vi "Initialize Motion.vi"(7 "Location":T1, 8 "error in":errorcluster, 9 "Bypass Motion Init":bool, 10 "Main Digitizer":T2=enum."NI Digitizer", 11 "Motion Settings In":T3={"No Motion?"=FALSE, "Motion System"=enum."MM3000", "Motion Bd ID"=0, "Motion Profile"="SMAC1", "# Axis"=0, "Reverse Z axis?"=FALSE, "SMAC Axis"=0, "scan pair"=enum."y-(x) scan", "RT fps"=0.0, "Steps per mm"=[], "Motor Parameters"={"velocity ct/s"=[], "accel ct/s^2"=[]}, "One Way Scan"=FALSE, "Reverse One Way Scan"=FALSE, "Global Position (mm)"=[], "Plane"=0, "Distance between\nscan lines (um)"=0.0, "Distance between\nscan planes (um)"=0.0, "number of scan planes"=0, "Total steps in line"=0, "Xtra plane\ndistance  (um)"=0, "Xtra planes "=0, "Add Axis"=FALSE, "overshoot cts"=0, "BKPT Shift"=0, "Scan Start Time (ms)"=0, "ESP VISA"="", "3rd Axis"=1, "GL Ref Out"=refnum, "Galil Address"=""} {"3rd Axis" items=["x", "y", "z", "w"]; "Xtra planes" min=1; "Xtra plane\ndistance  (um)" min=0; "Distance between\nscan planes (um)" format="%.2f"; "Distance between\nscan lines (um)" format="%.2f"; "SMAC Axis" items=["None"=0, "Axis 1"=1, "Axis 2"=2, "Axis 3"=3, "Axis 4"=4, "Axis 5"=5, "Axis 6"=6, "Axis 7"=7, "Axis 8"=8, "Vector Space 1"=17, "Vector Space 2"=18, "Vector Space 3"=19, "Vector Space 4"=20]; "Motion Bd ID" min=1 max=32 step=1}) -> (0 "error out":errorcluster, 1 "Initialization Failed!!":bool, 3 "Motion Settings":T3={"No Motion?"=FALSE, "Motion System"=enum."MM3000", "Motion Bd ID"=0, "Motion Profile"="SMAC1", "# Axis"=0, "Reverse Z axis?"=FALSE, "SMAC Axis"=0, "scan pair"=enum."y-(x) scan", "RT fps"=0.0, "Steps per mm"=[], "Motor Parameters"={"velocity ct/s"=[], "accel ct/s^2"=[]}, "One Way Scan"=FALSE, "Reverse One Way Scan"=FALSE, "Global Position (mm)"=[], "Plane"=0, "Distance between\nscan lines (um)"=0.0, "Distance between\nscan planes (um)"=0.0, "number of scan planes"=0, "Total steps in line"=0, "Xtra plane\ndistance  (um)"=0, "Xtra planes "=0, "Add Axis"=FALSE, "overshoot cts"=0, "BKPT Shift"=0, "Scan Start Time (ms)"=0, "ESP VISA"="", "3rd Axis"=1, "GL Ref Out"=refnum, "Galil Address"=""} {"3rd Axis" items=["x", "y", "z", "w"]; "Xtra planes" min=1; "Xtra plane\ndistance  (um)" min=0; "Distance between\nscan planes (um)" format="%.2f"; "Distance between\nscan lines (um)" format="%.2f"; "SMAC Axis" items=["None"=0, "Axis 1"=1, "Axis 2"=2, "Axis 3"=3, "Axis 4"=4, "Axis 5"=5, "Axis 6"=6, "Axis 7"=7, "Axis 8"=8, "Vector Space 1"=17, "Vector Space 2"=18, "Vector Space 3"=19, "Vector Space 4"=20]; "Motion Bd ID" min=1 max=32 step=1})   [LabVIEW 2022 SP3]
uses:
  NI_controller/-NI_MotionRoutines/MotionParameters.ctl
  NI_controller/-NI_MotionRoutines/MotionSys.ctl
  -MotionRoutines/ScanAxis.ctl
  -MotionRoutines/3rdAxis.ctl
  Digitizers/-DigitizerRoutines/Digitizer.ctl
  -ScanSystem/Controls/location.ctl
  Galil/Command Menu.ctl
  <vilib>/DAQmx/write.llb/DAQmx Write (Digital Bool 1Line 1Point).vi
  -MotionRoutines/MotionGlobals.vi
  <vilib>/DAQmx/miscellaneous.llb/DAQmx Fill In Error Info.vi
  <instrlib>/Newport ESP301/Newport ESP301.lvlib
panel:
  # "1-D and 2-D B scan settings"
  # "1-D and 2-D B scan settings"
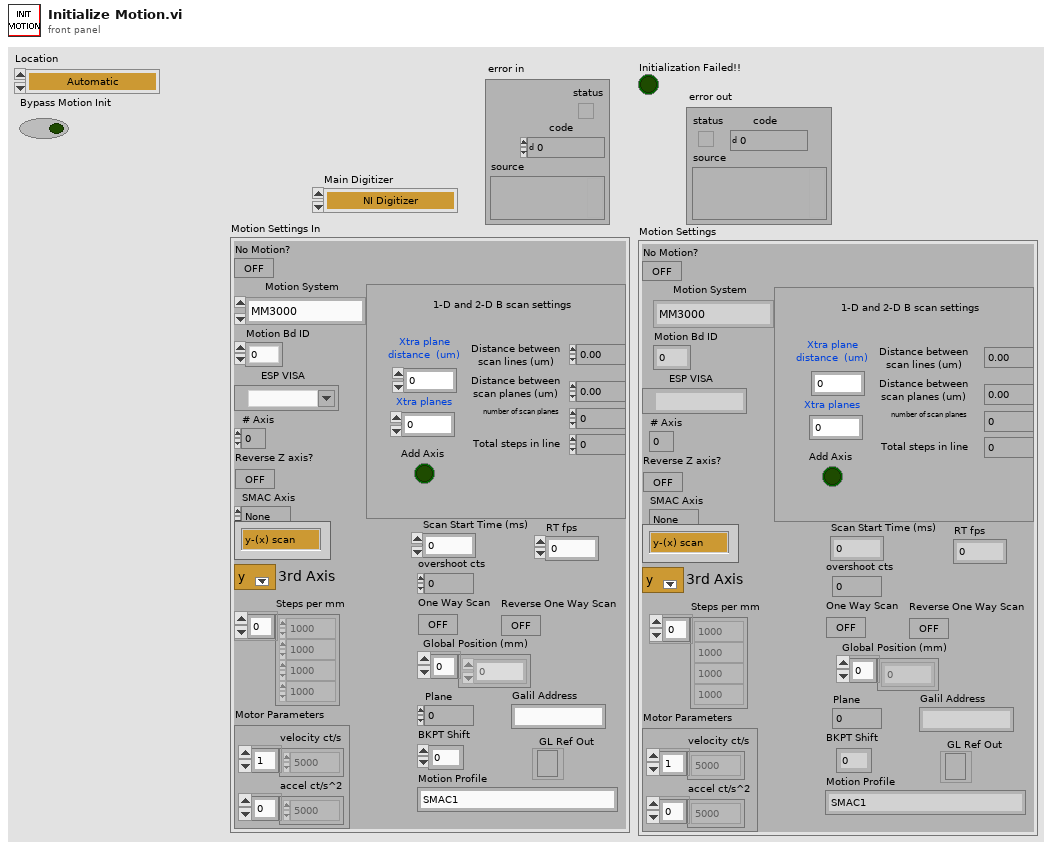
[diagram p1: front panel]
types:
  T1 = typedef "location.ctl" = enum16{"Automatic", "WCM Main", "Hawaii", "Columbia MM3000", "Columbia  NI System", "NYU", "RRI 2", "UHI Allen", "CUMC RT", "Chiba", "Stony Brook", "WCM Microscopy", "WCM Aeoretch", "WCM Optics Lab", "WCM Main 2Axis", "WCM Rotation", "WCM SAM SMAC", "SERI GP", "SERI SAM 2023"}
  T2 = typedef "Digitizer.ctl" = enum16{"Acqiris Digitizer", "NI Digitizer", "LeCroy", "GaGe", "AlazarTech", "No Digitizer", "Teledyne"}
  T3 = typedef "MotionParameters.ctl" = cluster{"No Motion?":bool, "Motion System":T4, "Motion Bd ID":u8, "Motion Profile":string, "# Axis":i8, "Reverse Z axis?":bool, "SMAC Axis":u16, "scan pair":T5, "RT fps":sgl, "Steps per mm":i32[], "Motor Parameters":cluster{"velocity ct/s":dbl[], "accel ct/s^2":dbl[]}, "One Way Scan":bool, "Reverse One Way Scan":bool, "Global Position (mm)":dbl[], "Plane":i32, "Distance between\nscan lines (um)":sgl, "Distance between\nscan planes (um)":sgl, "number of scan planes":i32, "Total steps in line":i32, "Xtra plane\ndistance  (um)":i32, "Xtra planes ":i32, "Add Axis":bool, "overshoot cts":i32, "BKPT Shift":i32, "Scan Start Time (ms)":u32, "ESP VISA":refnum<visa-resource-name>, "3rd Axis":T6, "GL Ref Out":refnum<k7>, "Galil Address":string}
  T4 = typedef "MotionSys.ctl" = enum16{"MM3000", "NI 735x", "Newport ESP", "No Motion Card", "Galil"}
  T5 = typedef "ScanAxis.ctl" = enum16{"y-(x) scan", "x-(y) scan", "z-(x) scan", "z-(y) scan", "y-(z) scan", "x-(z) scan", "w-(x) scan", "w-(y) scan", "w-(z) scan", "x-(w) scan", "y-(w) scan", "z-(w) scan"}
  T6 = typedef "3rdAxis.ctl" = u16
  T7 = cluster{"Port A (T:output, F:input)":bool, "Port B (T:output, F:input)":bool}
  T8 = typedef "Command Menu.ctl" = enum16{"CommandPassThrough", "Abort Motion", "Define Pos", "Velocity", "Acceleration", "Deceleration", "Position Rel", "Postion Abs", "Begin Move", "After Move", "Home", "KI", "KD", "KP", "IL", "Config I/O", "Set Bit", "Clear Bit", "Motor Off", "Moto On", "Status", "Execute", "Halt Execute", "HX Status", "Tell Velocity", "Check Motion", "BreakPoint", "Tell Position", "Current Code Line", "Tell Switches", "OC Force On", "OC Off", "Pos Soft Limit", "Rev Soft Limit"}
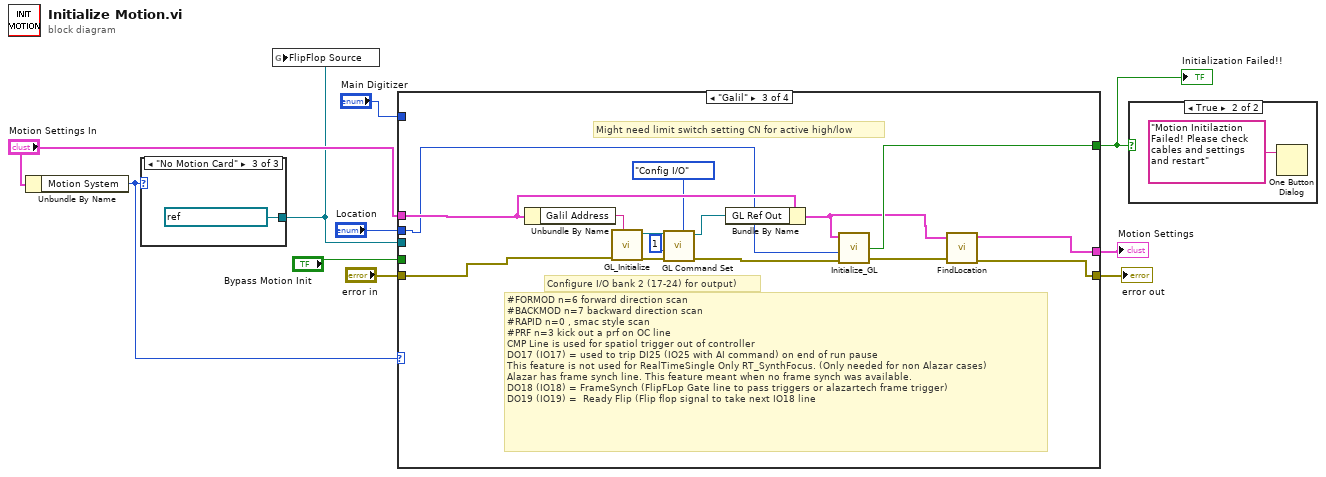
[diagram p0: block diagram]
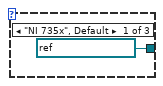
[diagram p3: hidden frame]
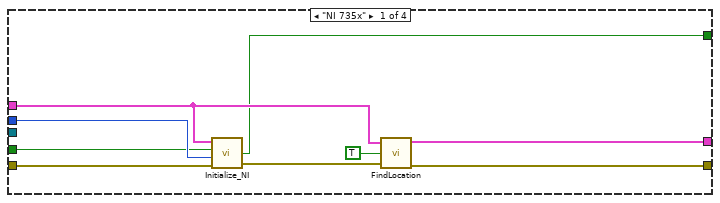
[diagram p5: hidden frame]
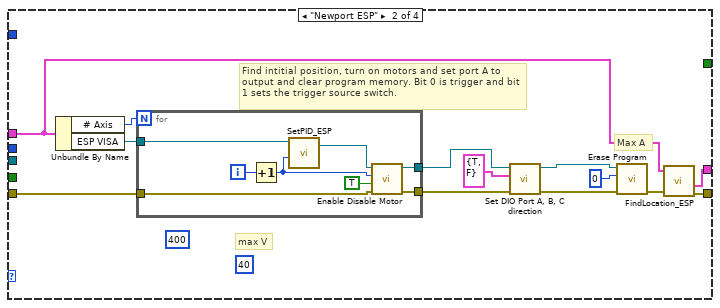
[diagram p6: hidden frame]
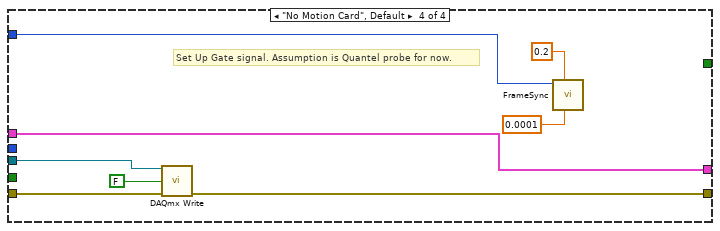
[diagram p7: hidden frame]
diagram:
  n1 = Unbundle By Name("Motion Settings In") -> ("Motion System"=w8:T4)
  n2 = case shown="\"No Motion Card\"" w8 {
    tunnel: [refnum<k21> "Dev1 FlipFlop" ("FlipFlop Source") _ refnum<k21> "QuantFlipFlop" ("FlipFlop Source")] -> w7
    frame "NI 735x", Default {
    }
    frame "Galil" {
    }
    frame "No Motion Card" {
    }
  }
  n3 = global write "MotionGlobals.vi" "FlipFlop Source"(w7) -> ()
  n4 = case shown="\"Galil\"" w8 {
    tunnel: w7 -> [_ _ _ w63]
    tunnel: "Motion Settings In" -> [w19 w26 w56 w61]
    tunnel: [w20 w28 w57 w61] -> w9
    tunnel: [w18 _ w46 _] -> w4
    tunnel: "error in" -> [w17 w22 w55 w59]
    tunnel: [w16 w24 w47 w60] -> w5
    tunnel: "Main Digitizer" -> [_ _ _ w58]
    tunnel: "Location" -> [w14 _ w54 _]
    tunnel: "Bypass Motion Init" -> [w13 _ _ _]
    frame "NI 735x" {
      n5 = call "Initialize_NI.vi"("Motion Settings"=w19, "Bypass Motion Init"=w13, "Location"=w14, "error in"=w17) -> ("Initialization Failed!!"=w18:bool, "error out"=w21:errorcluster)  [unwired: 1 in, 1 out]
      n6 = call "FindLocation.vi"("Motion Settings"=w19, "Wait for Motion Complete"=TRUE, "error in (no error)"=w21) -> ("Motion Settings Out"=w20:T3, "error out"=w16:errorcluster)  [unwired: 2 out]
    }
    frame "Newport ESP" {
      (unwired) 400
      (unwired) 40
      # "Max A"
      # "max V"
      # "Find intitial position, turn on motors and set port A to output and clear program memory. Bit 0 is trigger and bit 1 sets the trigger source switch."
      n7 = Unbundle By Name(w26) -> ("# Axis"=w25:i8, "ESP VISA"=w30:refnum<visa-resource-name>)
      n8 = for {
        N: w25 -> [_]
        tunnel: [w40] -> w29
        tunnel: w30 -> [w39]
        tunnel: [w36] -> w23
        tunnel: w22 -> [w35]
        i -> [w42]
        n9 = Increment(x=w42) -> (x+1=w37:i32)
        n10 = call "SetPID_ESP.vi"("VISA resource name"=w39, "Axis"=w37) -> ("VISA resource name out"=w38:refnum<visa-resource-name>)  [unwired: 4 in]
        n11 = call <instrlib>:"Enable Disable Motor.vi"("error in (no error)"=w35, "Action (OFF)"=TRUE, "Axis (1)"=w37, "VISA resource name"=w38) -> ("error out"=w36:errorcluster, "VISA resource name out"=w40:refnum<visa-resource-name>)  [unwired: 2 in]
      }
      n12 = call <instrlib>:"Set DIO Port A, B, C direction.vi"("error in (no error)"=w23, "Port A, B direction"=T7 {"Port A (T:output, F:input)"=TRUE, "Port B (T:output, F:input)"=FALSE}, "VISA resource name"=w29) -> ("error out"=w31:errorcluster, "VISA resource name out"=w32:refnum<visa-resource-name>)  [unwired: 7 in]
      n13 = call <instrlib>:"Erase Program.vi"("error in (no error)"=w31, "Program # (1)"=0, "VISA resource name"=w32) -> ("error out"=w27:errorcluster)  [unwired: 3 in, 1 out]
      n14 = call "FindLocation_ESP.vi"("Motion Settings"=w26, "error in (no error)"=w27) -> ("Motion Settings Out"=w28:T3, "error out"=w24:errorcluster)  [unwired: 1 in, 2 out]
    }
    frame "Galil" {
      # "Configure I/O bank 2 (17-24) for output)"
      # "#FORMOD n=6 forward direction scan\n#BACKMOD n=7 backward direction scan\n#RAPID n=0 , smac style scan\n#PRF n=3 kick out a prf on OC line\nCMP Line is used for spatiol trigger out of controller\nDO17 (IO17) = used to trip DI25 (IO25 with AI command) on end of run pause \nThis feature is not used for RealTimeSingle Only RT_SynthFocus. (Only needed for non Alazar cases)\nAlazar has frame synch line. This feature meant when no frame synch was available.\nDO18 (IO18) = FrameSynch (FlipFLop Gate line to pass triggers or alazartech frame trigger)\nDO19 (IO19) =  Ready Flip (Flip flop signal to take next IO18 line"
      # "Might need limit switch setting CN for active high/low"
      n15 = Unbundle By Name(w56) -> ("Galil Address"=w51:string)
      n16 = call "GL_Initialize.vi"("IP Address/COM"=w51, "error in (no error)"=w55) -> ("error out"=w49:errorcluster, "GL Ref Out"=w50:refnum<k7>)  [unwired: 4 in, 2 out]
      n17 = call "GL Command Set.vi"("Command"=Command_Menu."Config I/O", "error in (no error)"=w49, "Value"=1, "Galil.IGalil"=w50) -> ("error out"=w48:errorcluster, "ref out"=w45:refnum<k7>)  [unwired: 3 in, 3 out]
      n18 = Bundle By Name(cluster=w56, "GL Ref Out"=w45) -> (w43:T3)
      n19 = call "Initialize_GL.vi"("Motion Settings"=w43, "Location"=w54, "error in"=w48) -> ("Initialization Failed!!"=w46:bool, "error out"=w44:errorcluster)  [unwired: 2 in, 1 out]
      n20 = call "FindLocation.vi"("Motion Settings"=w43, "error in (no error)"=w44) -> ("Motion Settings Out"=w57:T3, "error out"=w47:errorcluster)  [unwired: 1 in, 2 out]
    }
    frame "No Motion Card", Default {
      # "Set Up Gate signal. Assumption is Quantel probe for now."
      n21 = call-poly <vilib>:"DAQmx Write.vi"("task/channels in"=w63, "data"=FALSE, "error in"=w59) -> ("error out"=w60:errorcluster)  [unwired: 10 in, 2 out]
      n22 = call "FrameSync.vi"("LowTime"=0.0001, "Gate Length"=0.2, "Main Digitizer"=w58) -> ()  [unwired: 7 in, 2 out]
    }
  }
  "Motion Settings" <- w9
  "Initialization Failed!!" <- w4
  "error out" <- w5
  n23 = case shown="True" w4 {
    frame False {
    }
    frame True {
      n24 = One Button Dialog(message="Motion Initilaztion Failed! Please check cables and settings and restart") -> ()  [unwired: 1 in, 1 out]
    }
  }
